vi "Test_Second_min.vi"() -> ()   [LabVIEW 2022 SP3]
panel:
  in  "stop":bool
  in  "Array":dbl[](array[numeric])
  out "AP3":dbl
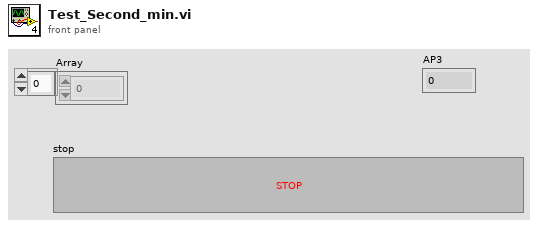
[diagram p1: front panel]
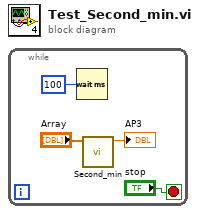
[diagram p0: block diagram]
diagram:
  n1 = while {
    stop <- "stop" stop-if-true
    n2 = Wait (ms)(milliseconds to wait=u32 100) -> ()  [unwired: 1 out]
    n3 = call "Second_min.vi"("Array"="Array") -> ("output"=→"AP3":dbl)  [unwired: 9 in, 1 out]
  }
